vi "Get Help.vi"() -> ()   [LabVIEW 2013, in "HadCon.lvlib"]
uses:
  <instrlib>/HadCon/HadCon.lvlib
panel:
  out "Help":string
  out "Error Out":errorcluster
  in  "VISA resource name":refnum<visa-resource-name>
  out "Instrument Firmware Revision":string
  out "Instrument Driver Revision":string
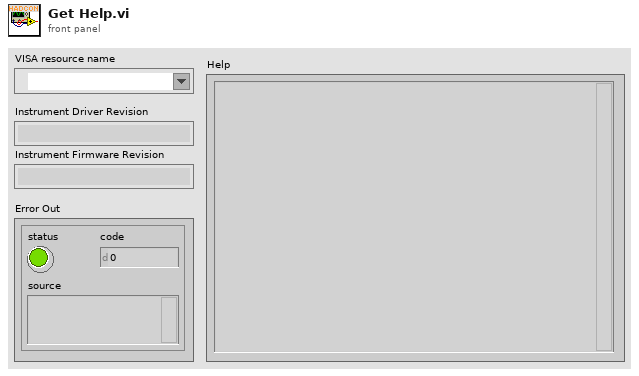
[diagram p1: front panel]
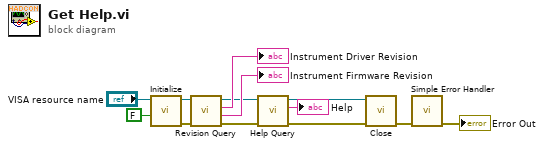
[diagram p0: block diagram]
diagram:
  n1 = call <instrlib>:"Initialize.vi"("Reset (True)"=FALSE, "VISA resource name"="VISA resource name") -> ("error out"=w12:errorcluster, "VISA resource name out"=w13:refnum<visa-resource-name>)  [unwired: 8 in]
  n2 = call <instrlib>:"Revision Query.vi"("error in (no error)"=w12, "VISA resource name"=w13) -> ("error out"=w5:errorcluster, "Instrument Firmware Revision"=→"Instrument Firmware Revision":string, "Instrument Driver Revision"=→"Instrument Driver Revision":string, "VISA resource name out"=w6:refnum<visa-resource-name>)  [unwired: 6 in]
  n3 = call <instrlib>:"Help Query.vi"("error in (no error)"=w5, "VISA resource name"=w6) -> ("error out"=w2:errorcluster, "Help"=→"Help":string, "VISA resource name out"=w3:refnum<visa-resource-name>)  [unwired: 7 in]
  n4 = call <instrlib>:"Close.vi"("error in (no error)"=w2, "VISA resource name"=w3) -> ("error out"=w9:errorcluster)  [unwired: 9 in]
  n5 = call <vilib>:"Simple Error Handler.vi"("error in (no error)"=w9) -> ("error out"=→"Error Out":errorcluster)  [unwired: 4 in, 4 out]
